vi "Set Header and Data.vi"(6 "Data Array":dbl[](array[numeric]), 8 "error in (no error)":errorcluster, 9 "Data & Time String":string, 10 "Header":string, 11 "Report":refnum<class "Report.lvclass">) -> (0 "error out":errorcluster, 3 "Report out":refnum<class "Report.lvclass">)   [LabVIEW 2011, in "Report.lvclass"]
doc: "This method is in the parent class and is used by the child classes. It sets the header and data for the object.\n\nAAL 9/09"
uses:
  Report.lvclass
  Report.lvclass/Report.ctl
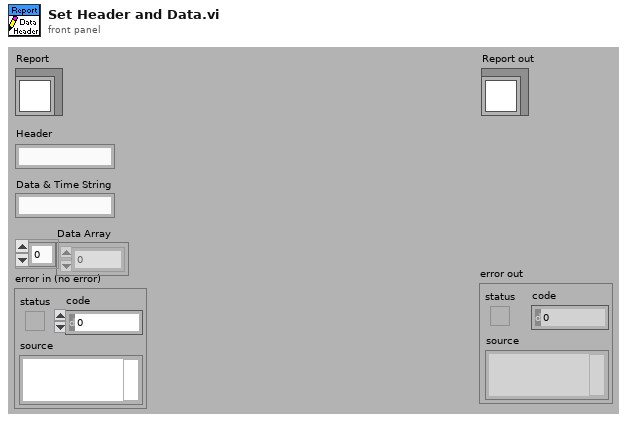
[diagram p1: front panel]
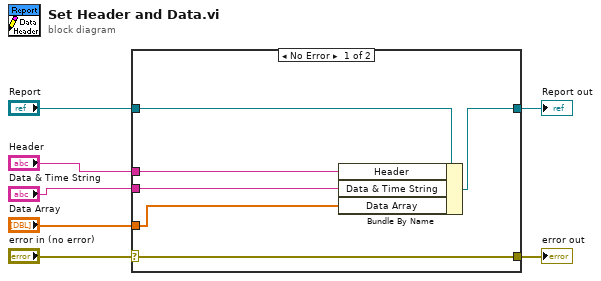
[diagram p0: block diagram]
diagram:
  n1 = case shown="No Error" "error in (no error)" {
    selector: "error in (no error)" -> [w13 w14]
    tunnel: [w13 w14] -> w6
    tunnel: [w11 w15] -> w4
    tunnel: "Report" -> [w12 w15]
    tunnel: "Header" -> [w10 _]
    tunnel: "Data & Time String" -> [w9 _]
    tunnel: "Data Array" -> [w8 _]
    frame No Error {
      n2 = Bundle By Name(cluster=w12, "Header"=w10, "Data & Time String"=w9, "Data Array"=w8) -> (w11:refnum<class "Report.lvclass">)
    }
    frame Error {
    }
  }
  "error out" <- w6
  "Report out" <- w4
